vi "Moving_Avg_Filter.vi"(7 "Coefficients":dbl[](array[numeric]), 11 "Input":dbl) -> (3 "Output":dbl, 6 "Moving Array":dbl[](array[numeric]))   [LabVIEW 2016]
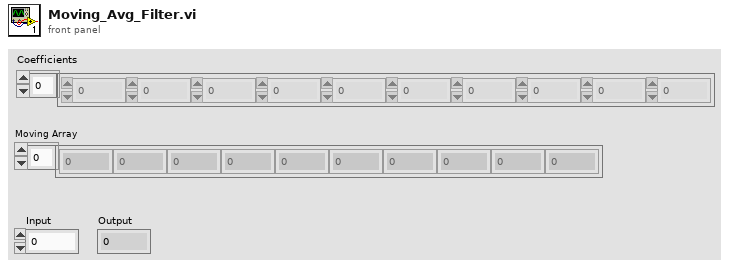
[diagram p1: front panel]
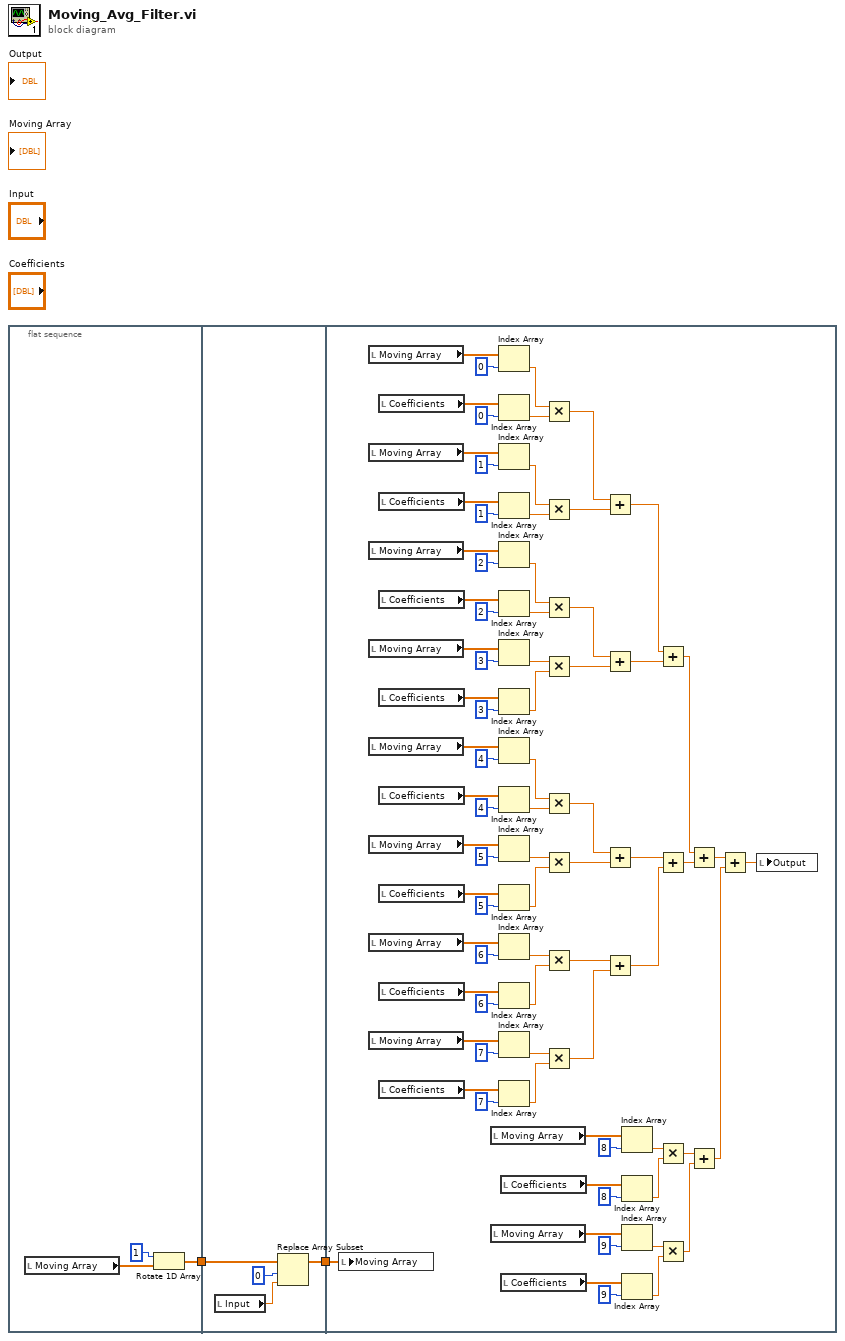
[diagram p0: block diagram]
diagram:
  n1 = flat-sequence {
    tunnel: [w3] -> w2
    tunnel: w2 -> [w8]
    tunnel: [w6] -> w1
    tunnel: w1 -> [w10]
    frame #0 {
      n2 = local read "Moving Array"() -> (w5:dbl[])
      n3 = Rotate 1D Array(1:w5, 2:1) -> (0:w3:dbl[])
    }
    frame #1 {
      n4 = local read "Input"() -> (w7:dbl)
      n5 = Replace Array Subset(array=w8, new element=w7, index=0) -> (w6:dbl[])
    }
    frame #2 {
      n6 = local write "Moving Array"(w10) -> ()
      n7 = local read "Moving Array"() -> (w88:dbl[])
      n8 = local read "Moving Array"() -> (w54:dbl[])
      n9 = local read "Moving Array"() -> (w82:dbl[])
      n10 = local read "Moving Array"() -> (w80:dbl[])
      n11 = local read "Moving Array"() -> (w84:dbl[])
      n12 = local read "Moving Array"() -> (w78:dbl[])
      n13 = local read "Moving Array"() -> (w56:dbl[])
      n14 = local read "Moving Array"() -> (w60:dbl[])
      n15 = local read "Coefficients"() -> (w86:dbl[])
      n16 = local read "Coefficients"() -> (w76:dbl[])
      n17 = local read "Coefficients"() -> (w74:dbl[])
      n18 = local read "Coefficients"() -> (w50:dbl[])
      n19 = local read "Coefficients"() -> (w52:dbl[])
      n20 = local read "Coefficients"() -> (w66:dbl[])
      n21 = local read "Coefficients"() -> (w64:dbl[])
      n22 = local read "Coefficients"() -> (w72:dbl[])
      n23 = local read "Moving Array"() -> (w58:dbl[])
      n24 = local read "Moving Array"() -> (w62:dbl[])
      n25 = Index Array(array=w88, index=0) -> (element=w49:dbl)
      n26 = Index Array(array=w86, index=0) -> (element=w48:dbl)
      n27 = Index Array(array=w54, index=1) -> (element=w47:dbl)
      n28 = Index Array(array=w76, index=1) -> (element=w46:dbl)
      n29 = Index Array(array=w82, index=2) -> (element=w45:dbl)
      n30 = Index Array(array=w74, index=2) -> (element=w44:dbl)
      n31 = Index Array(array=w80, index=3) -> (element=w43:dbl)
      n32 = Index Array(array=w50, index=3) -> (element=w42:dbl)
      n33 = Index Array(array=w84, index=4) -> (element=w41:dbl)
      n34 = Index Array(array=w52, index=4) -> (element=w40:dbl)
      n35 = Index Array(array=w78, index=5) -> (element=w39:dbl)
      n36 = Index Array(array=w66, index=5) -> (element=w38:dbl)
      n37 = Index Array(array=w56, index=6) -> (element=w37:dbl)
      n38 = Index Array(array=w64, index=6) -> (element=w36:dbl)
      n39 = Index Array(array=w60, index=7) -> (element=w35:dbl)
      n40 = Index Array(array=w72, index=7) -> (element=w34:dbl)
      n41 = local read "Coefficients"() -> (w70:dbl[])
      n42 = local read "Coefficients"() -> (w68:dbl[])
      n43 = Multiply(x=w49, y=w48) -> (x*y=w29:dbl)
      n44 = Multiply(x=w47, y=w46) -> (x*y=w28:dbl)
      n45 = Multiply(x=w45, y=w44) -> (x*y=w27:dbl)
      n46 = Multiply(x=w43, y=w42) -> (x*y=w26:dbl)
      n47 = Multiply(x=w41, y=w40) -> (x*y=w25:dbl)
      n48 = Multiply(x=w39, y=w38) -> (x*y=w24:dbl)
      n49 = Multiply(x=w37, y=w36) -> (x*y=w23:dbl)
      n50 = Multiply(x=w35, y=w34) -> (x*y=w22:dbl)
      n51 = Add(x=w29, y=w28) -> (x+y=w19:dbl)
      n52 = Add(x=w27, y=w26) -> (x+y=w18:dbl)
      n53 = Add(x=w25, y=w24) -> (x+y=w17:dbl)
      n54 = Add(x=w23, y=w22) -> (x+y=w16:dbl)
      n55 = Index Array(array=w58, index=8) -> (element=w33:dbl)
      n56 = Index Array(array=w70, index=8) -> (element=w32:dbl)
      n57 = Index Array(array=w62, index=9) -> (element=w31:dbl)
      n58 = Index Array(array=w68, index=9) -> (element=w30:dbl)
      n59 = Add(x=w19, y=w18) -> (x+y=w15:dbl)
      n60 = Add(x=w17, y=w16) -> (x+y=w14:dbl)
      n61 = Multiply(x=w33, y=w32) -> (x*y=w21:dbl)
      n62 = Multiply(x=w31, y=w30) -> (x*y=w20:dbl)
      n63 = Add(x=w15, y=w14) -> (x+y=w13:dbl)
      n64 = Add(x=w21, y=w20) -> (x+y=w12:dbl)
      n65 = Add(x=w13, y=w12) -> (x+y=w11:dbl)
      n66 = local write "Output"(w11) -> ()
    }
  }
